vi "Read configuration.vi"(8 "error in":errorcluster, 11 "Shared Memory editor node in":refnum<class "Shared Memory editor node.lvclass">) -> (0 "error out":errorcluster, 2 "configuration":refnum<class "NISE_CEF_serializable configuration.lvclass">, 3 "Shared Memory editor node out":refnum<class "Shared Memory editor node.lvclass">)   [LabVIEW 2013, in "Shared Memory editor node.lvclass"]
uses:
  Shared Memory editor node.lvclass
  <vilib>/NI/Configuration Framework/serializable configuration/NISE_CEF_serializable configuration.lvclass
  Shared Memory editor node.lvclass/Shared Memory editor node.ctl
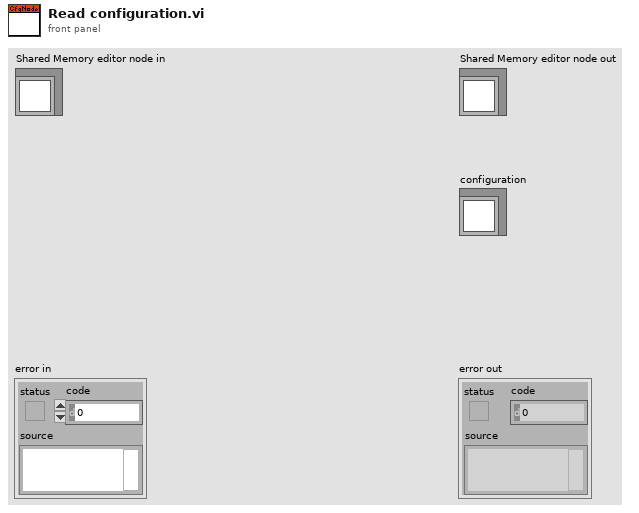
[diagram p1: front panel]
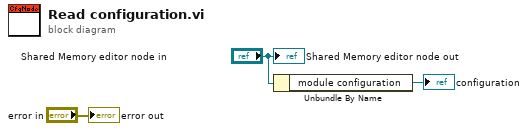
[diagram p0: block diagram]
diagram:
  n1 = Unbundle By Name("Shared Memory editor node in") -> ("module configuration"=→"configuration":refnum<class "Shared Memory configuration.lvclass">)
  "error out" <- "error in"
  "Shared Memory editor node out" <- "Shared Memory editor node in"
